vi "CAL-Probe Tube Cal Path (speaker).vi"(0 "Speaker":T1, 5 "Probe Tube Folder":path=path "C:/Data/Probe Tube Calibrations", 7 "Right":string, 9 "Left":string, 11 "error in (no error)":errorcluster) -> (6 "Probe Tube Cal Path":path, 15 "error out":errorcluster)   [LabVIEW 2020]
uses:
  Utility VIs/Type Defs/Speaker ring.ctl
  SubVIs/Calibration Globals.vi
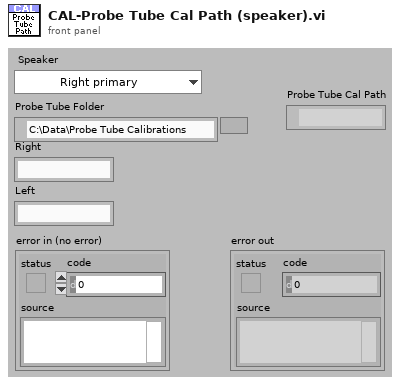
[diagram p1: front panel]
types:
  T1 = typedef "Speaker ring.ctl" = enum16{"Right primary", "Right secondary", "Left primary", "Left secondary"}
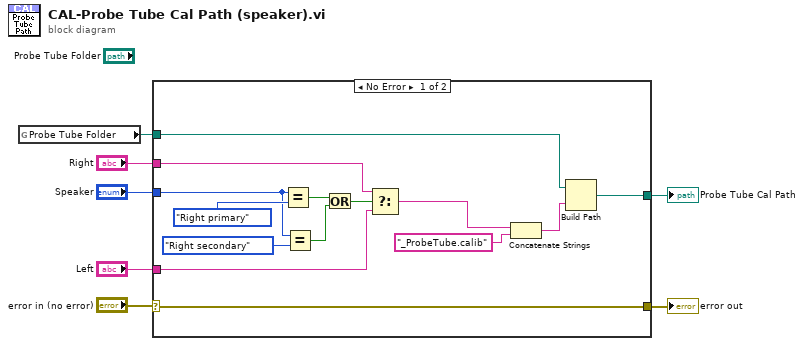
[diagram p0: block diagram]
diagram:
  n1 = global read "Calibration Globals.vi" "Probe Tube Folder"() -> (w1:path)
  n2 = case shown="No Error" "error in (no error)" {
    selector: "error in (no error)" -> [w8 w22]
    tunnel: "Speaker" -> [w19 _]
    tunnel: "Right" -> [w15 _]
    tunnel: "Left" -> [w14 _]
    tunnel: w1 -> [w11 _]
    tunnel: [w9 _] -> w3
    tunnel: [w8 w22] -> w2
    frame No Error {
      n3 = Equal?(x=w19, y=Speaker_ring."Right primary") -> (x = y?=w20:bool)
      n4 = Equal?(x=w19, y=Speaker_ring."Right secondary") -> (x = y?=w17:bool)
      n5 = Or(x=w20, y=w17) -> (x .or. y?=w16:bool)
      n6 = Select(t=w15, s=w16, f=w14) -> (s? t:f=w12:string)
      n7 = Concatenate Strings(w12, "_ProbeTube.calib" ("string")) -> (w10:string)
      n8 = Build Path(base path=w11, name or relative path=w10) -> (appended path=w9:path)
    }
    frame Error {
    }
  }
  "error out" <- w2
  "Probe Tube Cal Path" <- w3
